vi "EXCOM_26.vi"(0 "VISA resource name":refnum<visa-resource-name>) -> (1 "OK Done":bool=TRUE, 2 "STATL":bool[](array[boolean])=[TRUE, FALSE, FALSE, FALSE, FALSE, FALSE, FALSE, FALSE, FALSE, FALSE, FALSE, FALSE, FALSE, FALSE, FALSE, FALSE, FALSE, FALSE, FALSE, FALSE, FALSE, FALSE, FALSE, FALSE, FALSE, FALSE, FALSE, FALSE, FALSE, FALSE, FALSE, FALSE], 3 "STATH":bool[](array[boolean])=[FALSE, FALSE, TRUE, TRUE, FALSE, TRUE, TRUE, FALSE, FALSE, FALSE, FALSE, FALSE, FALSE, FALSE, FALSE, FALSE, FALSE, FALSE, FALSE, FALSE, FALSE, FALSE, FALSE, FALSE, FALSE, FALSE, FALSE, FALSE, FALSE, FALSE, FALSE, FALSE], 4 "STATLH":bool[](array[boolean]), 5 "STATEX":bool[](array[boolean]))   [LabVIEW 2010]
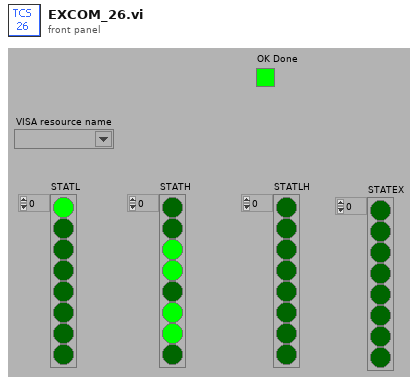
[diagram p1: front panel]
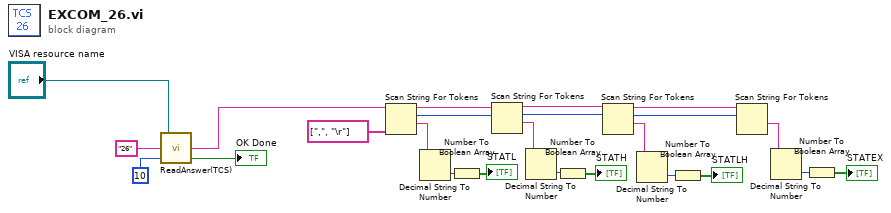
[diagram p0: block diagram]
diagram:
  n1 = call "ReadAnswer(TCS).vi"("Bytes to Read"=u32 10, "String to Send"="26", "VISA resource name"="VISA resource name") -> ("OK Done"=→"OK Done":bool, "String Received"=w23:string)  [unwired: 1 out]
  n2 = Scan String For Tokens(6:string[] [",", "\r"] ("delimiters (\\s,\\t,\\r,\\n)"), 9:w23) -> (1:w21:string, 2:w15:i32, 3:w17:string)  [unwired: 4 in, 1 out]
  n3 = Decimal String To Number(string=w21) -> (number=w13:i32)  [unwired: 2 in, 1 out]
  n4 = Number To Boolean Array(number=w13) -> (Boolean array=→"STATL":bool[])
  n5 = Scan String For Tokens(8:w15, 9:w17) -> (1:w19:string, 2:w14:i32, 3:w16:string)  [unwired: 4 in, 1 out]
  n6 = Decimal String To Number(string=w19) -> (number=w11:i32)  [unwired: 2 in, 1 out]
  n7 = Number To Boolean Array(number=w11) -> (Boolean array=→"STATH":bool[])
  n8 = Scan String For Tokens(8:w14, 9:w16) -> (1:w18:string, 2:w4:i32, 3:w3:string)  [unwired: 4 in, 1 out]
  n9 = Decimal String To Number(string=w18) -> (number=w10:i32)  [unwired: 2 in, 1 out]
  n10 = Number To Boolean Array(number=w10) -> (Boolean array=→"STATLH":bool[])
  n11 = Scan String For Tokens(8:w4, 9:w3) -> (1:w6:string)  [unwired: 4 in, 3 out]
  n12 = Decimal String To Number(string=w6) -> (number=w5:i32)  [unwired: 2 in, 1 out]
  n13 = Number To Boolean Array(number=w5) -> (Boolean array=→"STATEX":bool[])
